vi "ConvertTimes.vi"   [LabVIEW 2017, in "GP22_TDC_Arduinoed.lvlib"]
uses:
  GP22_TDC_Arduinoed.lvlib
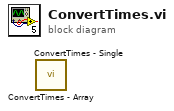
[diagram p0: block diagram]
diagram:
  n1 = call "ConvertTimes - Array.vi"() -> ()  [unwired: 1 in, 1 out]
  n2 = call "ConvertTimes - Single.vi"() -> ()  [unwired: 1 in, 1 out]
